vi "AJUSTE RPS.vi"() -> ()   [LabVIEW 2020]
panel:
  in  "Pérdidas":dbl(slide)=0.9 scale=0.0..1.0
  in  "Error":dbl(slide) step=1e-05 scale=-5.0..5.0
  in  "Stop Button":bool
  out "AJUSTE DE CURVAS":T1(graph)
  in  "Coeficientes de extinción":dbl[](array[slide]) step=1e-05 scale=-10.0..10.0
  in  "Número de capas":u32=1
  in  "Espesores (angstroms)":dbl[](array[slide]) scale=0.0..1000.0
  in  "Índices de refracción":dbl[](array[slide]) step=1e-05 scale=0.0..10.0
  in  "l(angstroms)":dbl=6328.0
  in  "File Path Control":path
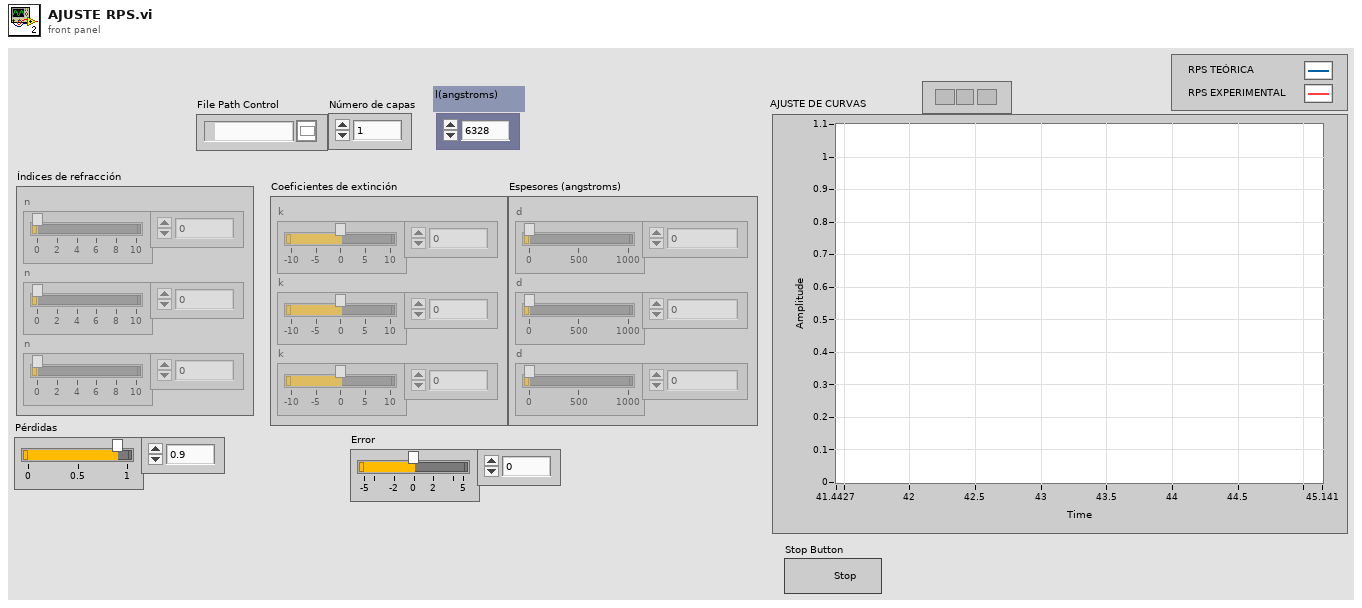
[diagram p1: front panel]
types:
  T1 = cluster{"EJE X":dbl[], "EJE Y NORMALIZADO":dbl[]}[]
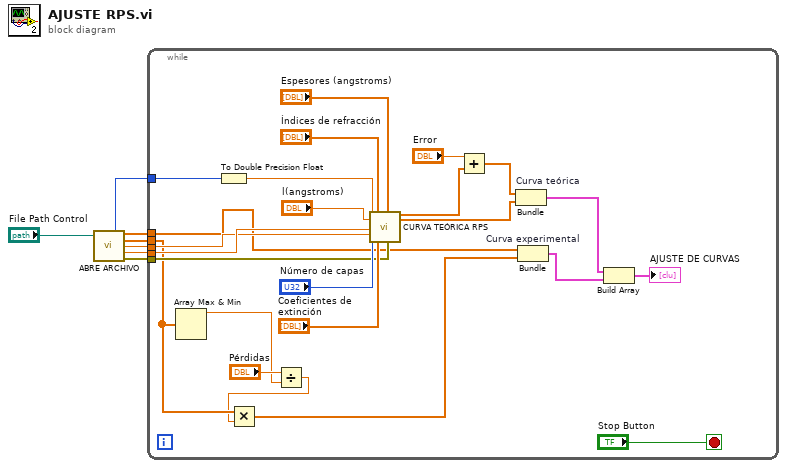
[diagram p0: block diagram]
diagram:
  n1 = call "ABRE ARCHIVO.vi"("File Path Control"="File Path Control") -> ("Número de datos"=w3:i32, "EJE X"=w2:dbl[], "EJE Y"=w1:dbl[], "Ángulo máximo"=w4:dbl, "Ángulo mínimo"=w5:dbl, "error out"=w6:errorcluster)  [unwired: 9 in]
  n2 = while {
    tunnel: w6 -> [w26]
    tunnel: w5 -> [w25]
    tunnel: w4 -> [w24]
    tunnel: w3 -> [w23]
    tunnel: w2 -> [w20]
    tunnel: w1 -> [w12]
    stop <- "Stop Button" stop-if-true
    n3 = Array Max & Min(array=w12) -> (max value=w10:dbl)  [unwired: 3 out]
    n4 = To Double Precision Float(number=w23) -> (double precision float=w22:dbl)
    n5 = Divide(x="Pérdidas", y=w10) -> (x/y=w9:dbl)
    n6 = Multiply(x=w12, y=w9) -> (x*y=w8:dbl[])
    n7 = call "CURVA TEÓRICA RPS.vi"("Resolución"=w22, "l(angstroms)"="l(angstroms)", "q mínimo"=w25, "q máximo"=w24, "Número de capas"="Número de capas", "Índices de refracción"="Índices de refracción", "Coeficientes de extinción"="Coeficientes de extinción", "Espesores (angstroms)"="Espesores (angstroms)", "error in (no error)"=w26) -> ("EJE X"=w14:dbl[], "EJE Y TEÓRICO"=w21:dbl[])  [unwired: 7 in, 2 out]
    n8 = Add(x="Error", y=w14) -> (x+y=w13:dbl[])
    n9 = Bundle "Curva teórica"(w13, "EJE Y TEÓRICO"=w21) -> (w19:cluster{dbl[], "EJE Y TEÓRICO":dbl[]})  [unwired: 1 in]
    n10 = Bundle "Curva experimental"("EJE X"=w20, w8) -> (w18:cluster{"EJE X":dbl[], dbl[]})  [unwired: 1 in]
    n11 = Build Array(w19, w18) -> (→"AJUSTE DE CURVAS":cluster{"EJE X":dbl[], "EJE Y TEÓRICO":dbl[]}[])
  }
